vi "Read configuration.vi"(8 "error in":errorcluster, 11 "cfg group in":refnum<class "cfg group.lvclass">) -> (0 "error out":errorcluster, 2 "configuration":refnum<class "NISE_CEF_serializable configuration.lvclass">, 3 "cfg group out":refnum<class "cfg group.lvclass">)   [LabVIEW 2013, in "cfg group.lvclass"]
uses:
  cfg group.lvclass
  CEF_TreeControl/serializable configuration/NISE_CEF_serializable configuration.lvclass
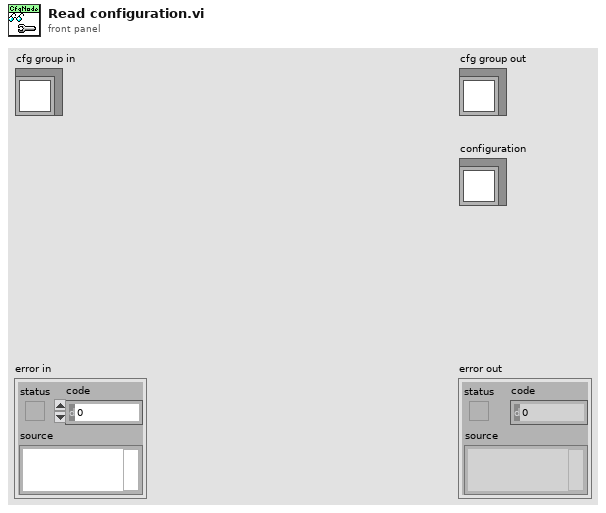
[diagram p1: front panel]
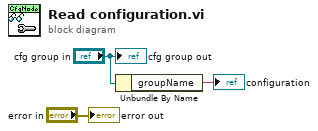
[diagram p0: block diagram]
diagram:
  n1 = Unbundle By Name("cfg group in") -> ("groupName"=→"configuration":string)
  "error out" <- "error in"
  "cfg group out" <- "cfg group in"
